vi "Low-Level Write.vi"(5 "Finished? (True)":bool=TRUE, 6 "Mask payload?":bool, 7 "Opcode (Text)":T1=1 items=["Cont. Frame"=0, "Text"=1, "Binary"=2, "Ping"=9, "Pong"=10], 8 "error in (no error)":errorcluster, 9 "timeout ms (5000)":i32=5000, 10 "Data":string, 11 "WebSockets in":refnum<class "WebSocket.lvclass">) -> (0 "error out":errorcluster, 3 "WebSockets out":refnum<class "WebSocket.lvclass">)   [LabVIEW 2013, in "WebSockets.lvlib" / "WebSocket.lvclass"]
doc: "Sends a WebSocket message to the client. Messages sent from the client must be masked but it is optional for the server.\n\nFinished should be set to True unless sending a fragmented message."
uses:
  WebSocket.lvclass
  Opcodes.ctl
panel:
  # "(leave as 'True' unless sending fragmented messages)"
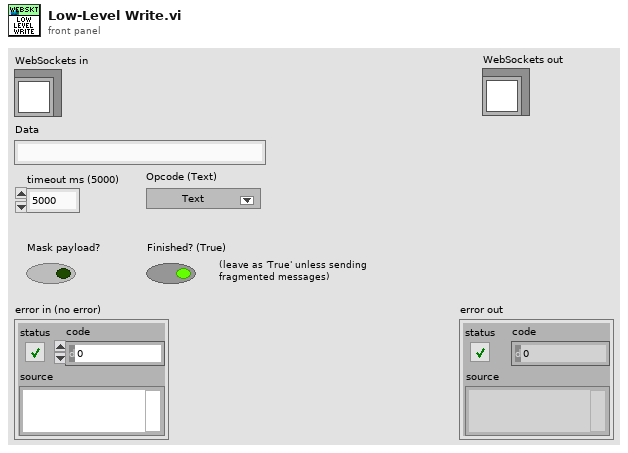
[diagram p1: front panel]
types:
  T1 = typedef "WebSockets.lvlib/WebSocket.lvclass/Opcodes.ctl" = u8
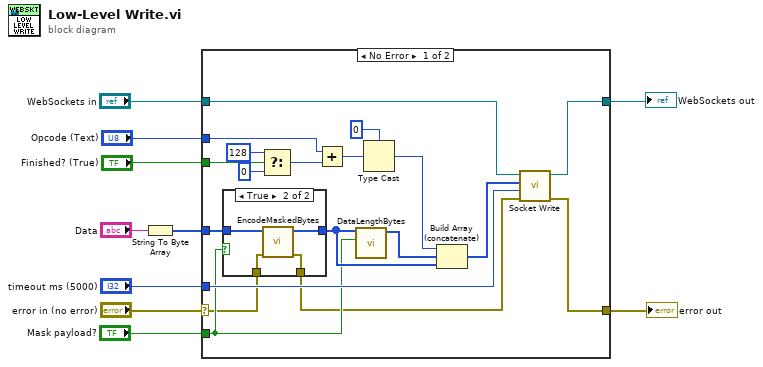
[diagram p0: block diagram]
diagram:
  n1 = String To Byte Array(string="Data") -> (unsigned byte array=w3:u8[])
  n2 = case shown="No Error" "error in (no error)" {
    selector: "error in (no error)" -> [w21 w37]
    tunnel: [w29 w37] -> w9
    tunnel: [w11 w36] -> w1
    tunnel: "WebSockets in" -> [w12 w36]
    tunnel: w3 -> [w24 _]
    tunnel: "timeout ms (5000)" -> [w25 _]
    tunnel: "Mask payload?" -> [w22 _]
    tunnel: "Finished? (True)" -> [w19 _]
    tunnel: "Opcode (Text)" -> [w17 _]
    frame No Error {
      n3 = case shown="True" w22 {
        tunnel: w24 -> [w31 w35]
        tunnel: [w31 w34] -> w23
        tunnel: w21 -> [w30 w33]
        tunnel: [w30 w32] -> w20
        frame False {
        }
        frame True {
          n4 = call "EncodeMaskedBytes.vi"("error in (no error)"=w33, "Raw Data"=w35) -> ("error out"=w32:errorcluster, "Masked Data"=w34:u8[])  [unwired: 8 in]
        }
      }
      n5 = Select(t=u8 128, s=w19, f=u8 0) -> (s? t:f=w18:u8)
      n6 = Add(x=w17, y=w18) -> (x+y=w27:T1)
      n7 = call "DataLengthBytes.vi"("Is masked?"=w22, "Data"=w23) -> ("Length Bytes"=w28:u8[])  [unwired: 9 in]
      n8 = Type Cast(type=u8 0 ("f"), x=w27) -> (*(type *) &x=w14:u8)
      n9 = Build Array (concatenate)(w14, w28, w23) -> (w26:u8[])
      n10 = call "Socket Write.vi"("error in (no error)"=w20, "timeout ms (5000)"=w25, "Bytes to write"=w26, "WebSocket in"=w12) -> ("error out"=w29:errorcluster, "WebSocket out"=w11:refnum<class "WebSocket.lvclass">)  [unwired: 5 in, 1 out]
    }
    frame Error {
    }
  }
  "error out" <- w9
  "WebSockets out" <- w1
